vi "test-create-path-trajectory-3-file.vi"() -> ()   [LabVIEW 2019]
uses:
  <vilib>/Rock Robotics/WPI/ThirdParty/MJansen/PathPlanner/TypeDef/PathPlannerTrajectory.ctl
  <vilib>/Rock Robotics/WPI/ThirdParty/MJansen/PathPlanner/TypeDef/PathPlannerTrajectoryState.ctl
  <vilib>/Rock Robotics/WPI/ThirdParty/JAS_Junk/TrajLib/TypeDef/TRANSLATION2D.ctl
  <vilib>/Rock Robotics/WPI/ThirdParty/JAS_Junk/TrajLib/TypeDef/ROTATION2D.ctl
  <vilib>/Rock Robotics/WPI/ThirdParty/MJansen/PathPlanner/TypeDef/PathPlannerPathConstraints.ctl
  <vilib>/Rock Robotics/WPI/ThirdParty/JAS_Junk/TrajLib/TypeDef/TRAJ_STATE.ctl
  <vilib>/Rock Robotics/WPI/ThirdParty/JAS_Junk/TrajLib/TypeDef/POSE2D.ctl
  <vilib>/Rock Robotics/WPI/ThirdParty/JAS_Junk/TrajLib/TypeDef/CHASSIS_SPEEDS.ctl
  <vilib>/Rock Robotics/WPI/ThirdParty/MJansen/PathPlanner/TypeDef/PathPlannerGoalEndState.ctl
  <vilib>/Rock Robotics/WPI/ThirdParty/MJansen/PathPlanner/TypeDef/PathPlannerPath.ctl
  <vilib>/Rock Robotics/WPI/ThirdParty/MJansen/PathPlanner/TypeDef/PathPlannerRotationTarget.ctl
  <vilib>/Rock Robotics/WPI/ThirdParty/MJansen/PathPlanner/TypeDef/PathPlannerConstraintsZone.ctl
  <vilib>/Rock Robotics/WPI/ThirdParty/MJansen/PathPlanner/TypeDef/PathPlannerEventMarker.ctl
  <vilib>/Rock Robotics/WPI/ThirdParty/MJansen/PathPlanner/TypeDef/PathPlannerCommandUtil.ctl
  <vilib>/Rock Robotics/WPI/ThirdParty/MJansen/PathPlanner/ENum/PathPlanner_CommandUtilType_ENUM.ctl
  <vilib>/Rock Robotics/WPI/ThirdParty/MJansen/PathPlanner/TypeDef/PathPlannerPathPoint.ctl
  <vilib>/Rock Robotics/WPI/ThirdParty/MJansen/PathPlanner/TypeDef/PathPlannerWaypoint.ctl
  <vilib>/Rock Robotics/WPI/ThirdParty/MJansen/PathPlanner/TypeDef/PathPlannerPointTowardsZone.ctl
  <vilib>/Rock Robotics/WPI/ThirdParty/MJansen/PathPlanner/TypeDef/PathPlannerIdealStartingState.ctl
  <vilib>/Rock Robotics/WPI/ThirdParty/JAS_Junk/TrajLib/Conv_Deg_Radians.vi
  <vilib>/Rock Robotics/WPI/ThirdParty/JAS_Junk/TrajLib/Rotation2d_CreateAngle.vi
  <vilib>/Rock Robotics/WPI/ThirdParty/MJansen/PathPlanner/VI/PathPlanner_Waypoint_AutoCtrlPoints.vi
  <vilib>/Rock Robotics/WPI/ThirdParty/JAS_Junk/TrajLib/Pose2d_getTranslation.vi
  <vilib>/Rock Robotics/WPI/ThirdParty/JAS_Junk/TrajLib/Pose2d_getRotation.vi
  <vilib>/Rock Robotics/WPI/ThirdParty/JAS_Junk/TrajLib/Translation2d_Minus.vi
  <vilib>/Rock Robotics/WPI/ThirdParty/JAS_Junk/TrajLib/Translation2d_Create_DistAng.vi
  <vilib>/Rock Robotics/WPI/ThirdParty/JAS_Junk/TrajLib/Translation2d_GetDistance.vi
  <vilib>/Rock Robotics/WPI/ThirdParty/MJansen/PathPlanner/VI/PathPlanner_Waypoint_AutoCtrlDistFactor.vi
  <vilib>/Rock Robotics/WPI/ThirdParty/JAS_Junk/TrajLib/Translation2d_Plus.vi
  <vilib>/Rock Robotics/WPI/ThirdParty/JAS_Junk/TrajLib/Translation2d_Create.vi
  <vilib>/Rock Robotics/WPI/ThirdParty/JAS_Junk/TrajLib/Rotation2d_GetAngleCosSin.vi
  <vilib>/Rock Robotics/WPI/ThirdParty/JAS_Junk/TrajLib/Util_CalcDist.vi
  <vilib>/Rock Robotics/WPI/ThirdParty/MJansen/PathPlanner/PathPlanner24.lvlib
  <vilib>/Rock Robotics/WPI/ThirdParty/JAS_Junk/TrajLib/Trajectory_Library.lvlib
  <vilib>/Rock Robotics/WPI/ThirdParty/MJansen/PathPlanner/TypeDef/PathPlannerTrajectoryEvent.ctl
  <vilib>/Rock Robotics/WPI/ThirdParty/MJansen/PathPlanner/TypeDef/PathPlannerTrajectoryEvents.ctl
panel:
  in  "Tab Control":T1(tab)
  in  "Output Trajectory File Name":string="C:\\Shares\\github\\PathPlannerLabVIEW\\PathPlannerSandbox24\\PathPlannerTestPath\\jim1.csv"
  in  "Position 1":T2={"TRANSLATION"={"X"=1.0, "Y"=1.0}, "ROTATION"={"VALUE"=0.0, "COS"=1.0, "SIN"=0.0}} {"ROTATION"."SIN" format="%13.4f"; "ROTATION"."COS" format="%13.4f"; "ROTATION"."VALUE" format="%13.4f"; "TRANSLATION"."Y" format="%14.3f"; "TRANSLATION"."X" format="%14.3f"}
  in  "Position 2":T2={"TRANSLATION"={"X"=1.3, "Y"=1.0}, "ROTATION"={"VALUE"=0.0, "COS"=1.0, "SIN"=0.0}} {"ROTATION"."SIN" format="%13.4f"; "ROTATION"."COS" format="%13.4f"; "ROTATION"."VALUE" format="%13.4f"; "TRANSLATION"."Y" format="%14.3f"; "TRANSLATION"."X" format="%14.3f"}
  in  "Position 3":T2={"TRANSLATION"={"X"=4.0, "Y"=3.7}, "ROTATION"={"VALUE"=1.57, "COS"=0.0, "SIN"=1.0}} {"ROTATION"."SIN" format="%13.4f"; "ROTATION"."COS" format="%13.4f"; "ROTATION"."VALUE" format="%13.4f"; "TRANSLATION"."Y" format="%14.3f"; "TRANSLATION"."X" format="%14.3f"}
  in  "Position 4":T2={"TRANSLATION"={"X"=4.0, "Y"=4.0}, "ROTATION"={"VALUE"=1.57, "COS"=0.0, "SIN"=1.0}} {"ROTATION"."SIN" format="%13.4f"; "ROTATION"."COS" format="%13.4f"; "ROTATION"."VALUE" format="%13.4f"; "TRANSLATION"."Y" format="%14.3f"; "TRANSLATION"."X" format="%14.3f"}
  in  "stop":bool
  in  "StartingSpeeds":T5 {"vOmega" format="%10.3f"; "vY" format="%10.3f"; "vX" format="%10.3f"}
  out "Error":bool
  out "Error 2":bool
  out "PathPlannerConstraints":T6={"MaxVelocityMps;"=0.0, "MaxAccelerationMpsSq;"=0.0, "MaxAngularVelRadPsEc;"=0.0, "MaxAngularAccRadPSecSq"=0.0, "Exists"=FALSE, "Unlimited"=FALSE, "NominalVoltageVolts"=12.0}
  out "GoalEndState":T7={"VelocityMPS"=0.0, "Rotation"={"VALUE"=0.0, "COS"=1.0, "SIN"=0.0}} {"Rotation"."SIN" format="%13.4f"; "Rotation"."COS" format="%13.4f"; "Rotation"."VALUE" format="%13.4f"}
  in  "Angle_Degrees":dbl=90.0
  in  "Velocity":dbl format="%#_13g"
  out "file read\nerror out":errorcluster
  in  "Input Path FileName":string="C:\\Shares\\github\\PathPlannerLabVIEW\\PathPlannerSandbox24\\PathPlannerTestPath\\jim1.path"
  out "write csv file\nerror out":errorcluster
  out "PathPlannerPath":T8={"Reversed"=FALSE, "RotationTargets"=[], "ConstraintZones"=[], "EventMarkers"=[], "GlobalConstraints"={"MaxVelocityMps;"=0.0, "MaxAccelerationMpsSq;"=0.0, "MaxAngularVelRadPsEc;"=0.0, "MaxAngularAccRadPSecSq"=0.0, "Exists"=FALSE, "Unlimited"=FALSE, "NominalVoltageVolts"=1.0}, "GoalEndState"={"VelocityMPS"=0.0, "Rotation"={"VALUE"=0.0, "COS"=1.0, "SIN"=0.0}}, "AllPoints"=[], "Name"="", "Waypoints"=[], "PointTowardsZones"=[], "IdealStartingState"={"VelocityMPS"=0.0, "Rotation"={"VALUE"=0.0, "COS"=1.0, "SIN"=0.0}}, "IsChoreoPath"=FALSE, "PreventFlipping"=FALSE} {"IdealStartingState"."Rotation"."SIN" format="%13.4f"; "IdealStartingState"."Rotation"."COS" format="%13.4f"; "IdealStartingState"."Rotation"."VALUE" format="%13.4f"; "PointTowardsZones"."TargetPosition"."Y" format="%14.3f"; "PointTowardsZones"."TargetPosition"."X" format="%14.3f"; "PointTowardsZones"."RotationOffset"."SIN" format="%13.4f"; "PointTowardsZones"."RotationOffset"."COS" format="%13.4f"; "PointTowardsZones"."RotationOffset"."VALUE" format="%13.4f"; "Waypoints"."nextControl"."Y" format="%14.3f"; "Waypoints"."nextControl"."X" format="%14.3f"; "Waypoints"."anchor"."Y" format="%14.3f"; "Waypoints"."anchor"."X" format="%14.3f"; "Waypoints"."prevControl"."Y" format="%14.3f"; "Waypoints"."prevControl"."X" format="%14.3f"; "AllPoints"."RotationTarget"."rotation"."SIN" format="%13.4f"; "AllPoints"."RotationTarget"."rotation"."COS" format="%13.4f"; "AllPoints"."RotationTarget"."rotation"."VALUE" format="%13.4f"; "AllPoints"."Position"."Y" format="%14.3f"; "AllPoints"."Position"."X" format="%14.3f"; "GoalEndState"."Rotation"."SIN" format="%13.4f"; "GoalEndState"."Rotation"."COS" format="%13.4f"; "GoalEndState"."Rotation"."VALUE" format="%13.4f"; "RotationTargets"."rotation"."SIN" format="%13.4f"; "RotationTargets"."rotation"."COS" format="%13.4f"; "RotationTargets"."rotation"."VALUE" format="%13.4f"}
  out "PathPlannerTrajectory":T18 {"States"."TargetHolonomicRotation"."SIN" format="%13.4f"; "States"."TargetHolonomicRotation"."COS" format="%13.4f"; "States"."TargetHolonomicRotation"."VALUE" format="%13.4f"; "States"."Heading"."SIN" format="%13.4f"; "States"."Heading"."COS" format="%13.4f"; "States"."Heading"."VALUE" format="%13.4f"; "States"."PositionMeters"."Y" format="%14.3f"; "States"."PositionMeters"."X" format="%14.3f"}
  out "outPathPlannerStates":T19[](array[typedef]) {"TargetHolonomicRotation"."SIN" format="%13.4f"; "TargetHolonomicRotation"."COS" format="%13.4f"; "TargetHolonomicRotation"."VALUE" format="%13.4f"; "Heading"."SIN" format="%13.4f"; "Heading"."COS" format="%13.4f"; "Heading"."VALUE" format="%13.4f"; "PositionMeters"."Y" format="%14.3f"; "PositionMeters"."X" format="%14.3f"}
  out "PathPlannerTrajectoryEvents":T20
  in  "Down Button":bool
  in  "Up Button":bool
  in  "index":i32 step=20
  out "LabVIEWStateCount":i32
  out "LabVIEWStates":T22[](array[typedef]) {"POSE"."ROTATION"."SIN" format="%13.4f"; "POSE"."ROTATION"."COS" format="%13.4f"; "POSE"."ROTATION"."VALUE" format="%13.4f"; "POSE"."TRANSLATION"."Y" format="%14.3f"; "POSE"."TRANSLATION"."X" format="%14.3f"}
  out "XY SPLINE":cluster{dbl[], dbl[]}[](graph)
  out "XY Graph":cluster{dbl[], dbl[]}[](graph)
  out "Sample Graph":dbl[][](graph)
  out "LabVIEW Time Plot":cluster{dbl[], dbl[]}[](graph)
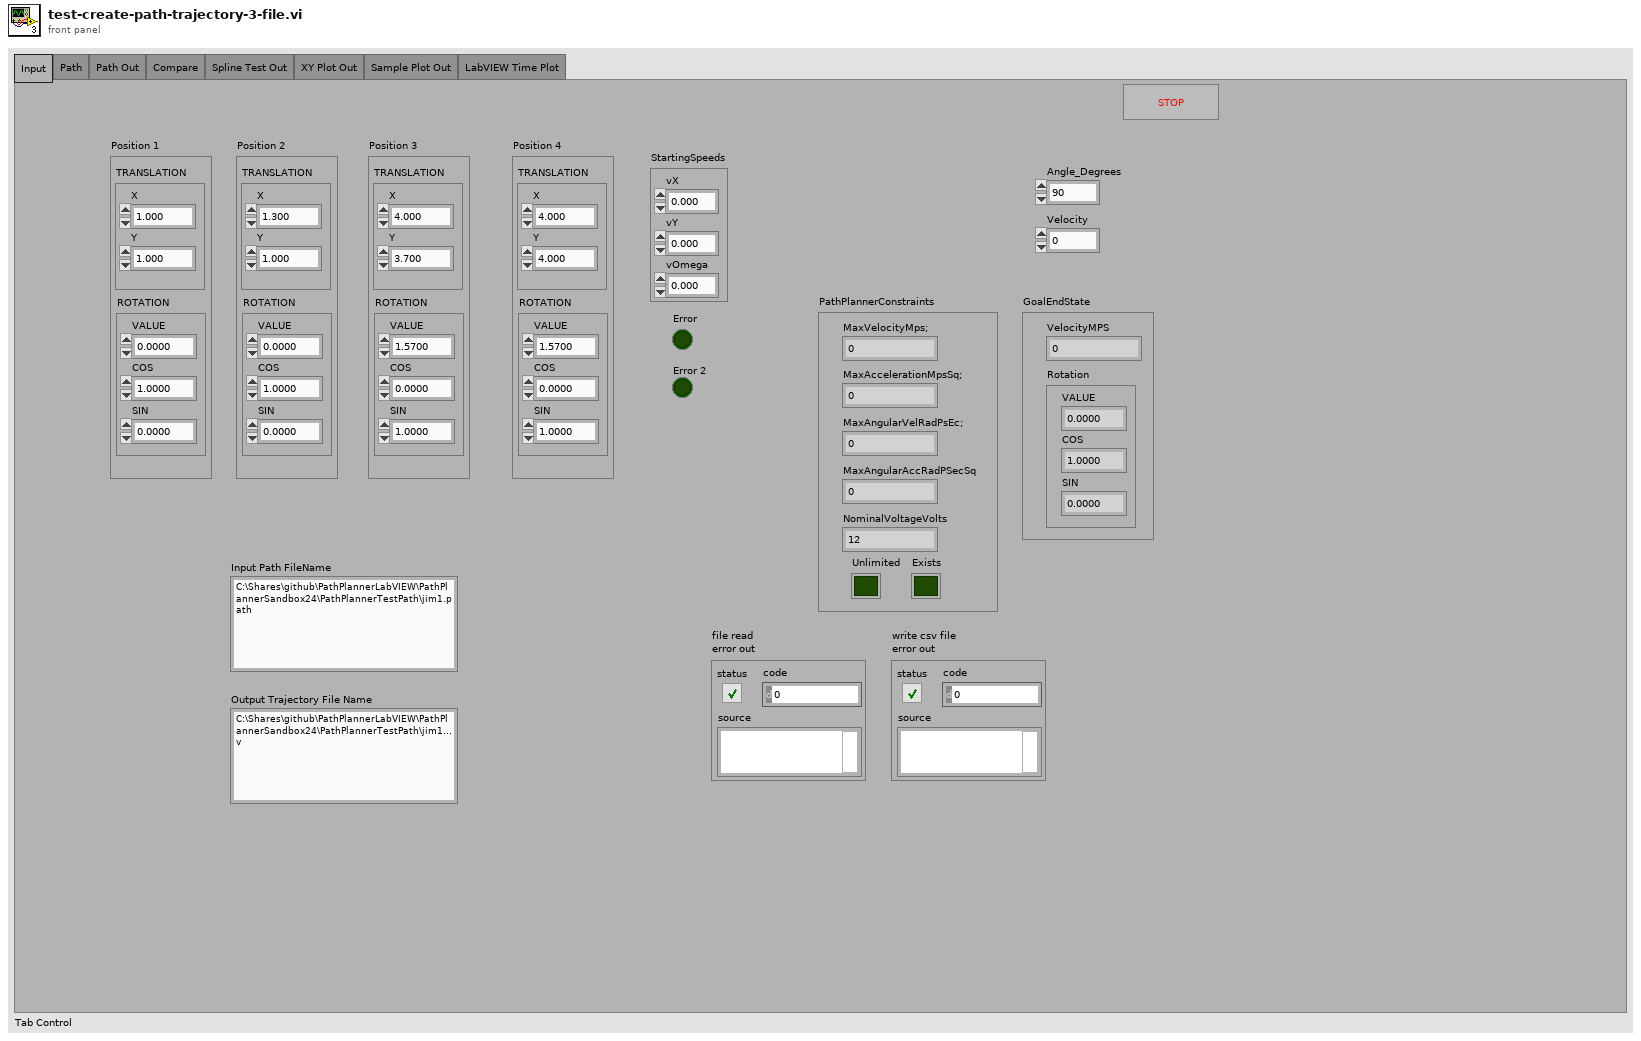
[diagram p1: front panel]
types:
  T1 = enum32{"Input", "Path", "Path Out", "Compare", "Spline Test Out", "XY Plot Out", "Sample Plot Out", "LabVIEW Time Plot"}
  T2 = typedef "Trajectory_Library.lvlib/POSE2D.ctl" = cluster{"TRANSLATION":T3, "ROTATION":T4}
  T3 = typedef "Trajectory_Library.lvlib/TRANSLATION2D.ctl" = cluster{"X":dbl, "Y":dbl}
  T4 = typedef "Trajectory_Library.lvlib/ROTATION2D.ctl" = cluster{"VALUE":dbl, "COS":dbl, "SIN":dbl}
  T5 = typedef "Trajectory_Library.lvlib/CHASSIS_SPEEDS.ctl" = cluster{"vX":dbl, "vY":dbl, "vOmega":dbl}
  T6 = typedef "PathPlanner24.lvlib/PathPlannerPathConstraints.ctl" = cluster{"MaxVelocityMps;":dbl, "MaxAccelerationMpsSq;":dbl, "MaxAngularVelRadPsEc;":dbl, "MaxAngularAccRadPSecSq":dbl, "Exists":bool, "Unlimited":bool, "NominalVoltageVolts":dbl}
  T7 = typedef "PathPlanner24.lvlib/PathPlannerGoalEndState.ctl" = cluster{"VelocityMPS":dbl, "Rotation":T4}
  T8 = typedef "PathPlanner24.lvlib/PathPlannerPath.ctl" = cluster{"Reversed":bool, "RotationTargets":T9[], "ConstraintZones":T10[], "EventMarkers":T11[], "GlobalConstraints":T6, "GoalEndState":T7, "AllPoints":T14[], "Name":string, "Waypoints":T15[], "PointTowardsZones":T16[], "IdealStartingState":T17, "IsChoreoPath":bool, "PreventFlipping":bool}
  T9 = typedef "PathPlanner24.lvlib/PathPlannerRotationTarget.ctl" = cluster{"position":dbl, "rotation":T4, "Exists":bool}
  T10 = typedef "PathPlanner24.lvlib/PathPlannerConstraintsZone.ctl" = cluster{"minPosition":dbl, "maxPosition":dbl, "Constraints":T6, "Present":bool}
  T11 = typedef "PathPlanner24.lvlib/PathPlannerEventMarker.ctl" = cluster{"Position":dbl, "Command":T12, "TriggerName":string, "EndPosition":dbl}
  T12 = typedef "PathPlanner24.lvlib/PathPlannerCommandUtil.ctl" = cluster{"waitTime":dbl, "name":string, "pathName":string, "commands":cluster{"type":T13, "waitTime":dbl, "name":string, "pathName":string}[], "type":T13}
  T13 = typedef "PathPlanner24.lvlib/PathPlanner_CommandUtilType_ENUM.ctl" = enum16{"Unknown", "Wait", "Named", "Path", "Sequential", "Parallel", "Race", "Deadline"}
  T14 = typedef "PathPlanner24.lvlib/PathPlannerPathPoint.ctl" = cluster{"Position":T3, "DistAlongPath":dbl, "MaxV":dbl, "Constraints":T6, "RotationTarget":T9, "WaypointRelativePos":dbl}
  T15 = typedef "PathPlanner24.lvlib/PathPlannerWaypoint.ctl" = cluster{"prevControl":T3, "anchor":T3, "nextControl":T3, "PrevExists":bool, "NextExists":bool}
  T16 = typedef "PathPlanner24.lvlib/PathPlannerPointTowardsZone.ctl" = cluster{"RotationOffset":T4, "Name":string, "TargetPosition":T3, "MinPosition":dbl, "MaxPosition":dbl}
  T17 = typedef "PathPlanner24.lvlib/PathPlannerIdealStartingState.ctl" = cluster{"VelocityMPS":dbl, "Rotation":T4}
  T18 = typedef "PathPlanner24.lvlib/PathPlannerTrajectory.ctl" = cluster{"States":T19[]}
  T19 = typedef "PathPlanner24.lvlib/PathPlannerTrajectoryState.ctl" = cluster{"TimeSeconds":dbl, "VelocityMPS":dbl, "AccerationMpsSq":dbl, "HeadingAngularVelRadPerSec":dbl, "PositionMeters":T3, "Heading":T4, "TargetHolonomicRotation":T4, "CurvatureRadPerMeter":dbl, "PathPlannerConstraints":T6, "DeltaPos":dbl, "WaypointRelPos":dbl}
  T20 = typedef "PathPlanner24.lvlib/PathPlannerTrajectoryEvents.ctl" = cluster{"EventCommands":T21[]}
  T21 = typedef "PathPlanner24.lvlib/PathPlannerTrajectoryEvent.ctl" = cluster{"TimeStampSec":dbl, "CommandUtil":T12}
  T22 = typedef "Trajectory_Library.lvlib/TRAJ_STATE.ctl" = cluster{"TimeSeconds":dbl, "Velocity":dbl, "Acceleration":dbl, "POSE":T2, "Curvature":dbl}
  T23 = typedef "Trajectory_Library.lvlib/TRAJECTORY.ctl" = cluster{"TotalTImeSecs":dbl, "States":T22[]}
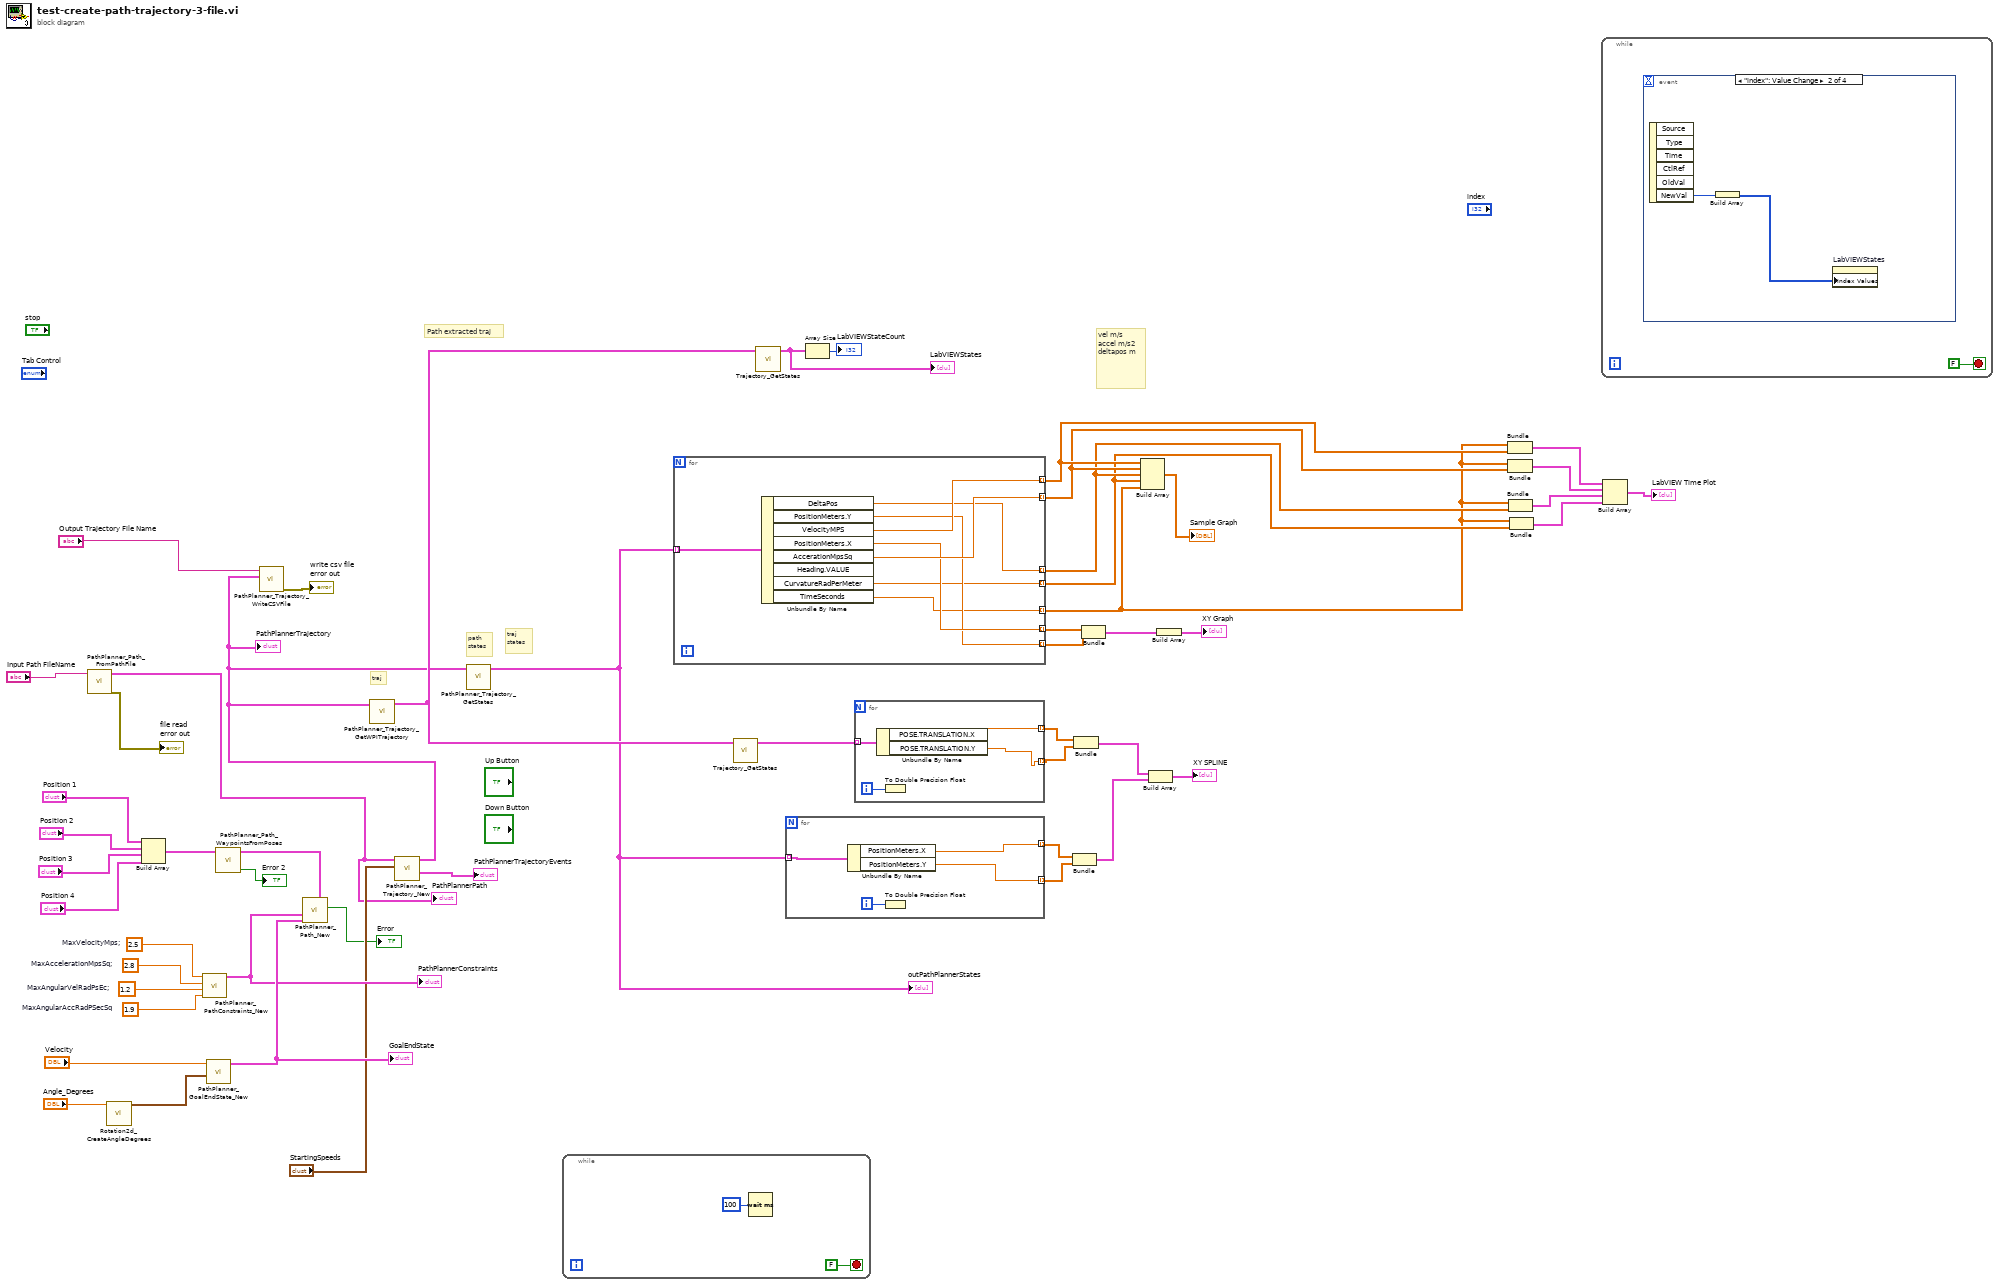
[diagram p0: block diagram]
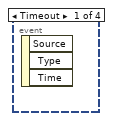
[diagram p2: hidden frame]
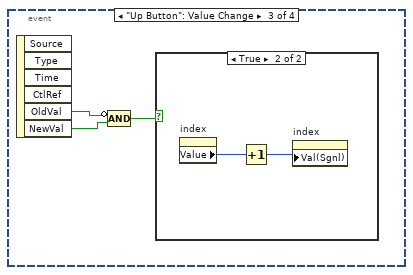
[diagram p3: hidden frame]
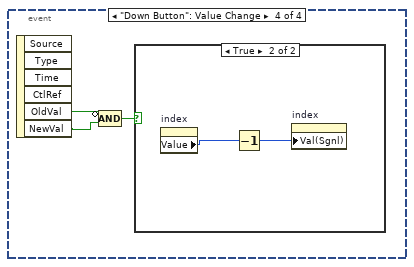
[diagram p5: hidden frame]
diagram:
  w15 = 2.5  # MaxVelocityMps;
  w16 = 2.8  # MaxAccelerationMpsSq;
  w17 = 1.2  # MaxAngularVelRadPsEc;
  w14 = 1.9  # MaxAngularAccRadPSecSq
  # "vel m/s\naccel m/s2\ndeltapos m"
  # "Path extracted traj"
  # "traj"
  # "traj\nstates"
  # "path\nstates"
  n1 = call <vilib>:"PathPlanner_Path_FromPathFile.vi"("FileName"="Input Path FileName") -> ("error out"=→"file read\nerror out":errorcluster, "PathPlannerPath"=w8:T8)  [unwired: 7 in, 2 out]
  "PathPlannerPath" <- w8
  n2 = call <vilib>:"Rotation2d_CreateAngleDegrees.vi"("Angle_Degrees"="Angle_Degrees") -> ("ROTATION"=w9:T4)  [unwired: 10 in]
  n3 = Build Array("Position 1", "Position 2", "Position 3", "Position 4") -> (w21:T2[])
  n4 = call <vilib>:"PathPlanner_PathConstraints_New.vi"("MaxAngularAccRadPSecSq"=w14, "MaxAngularVelRadPsEc;"=w17, "MaxAccelerationMpsSq;"=w16, "MaxVelocityMps;"=w15) -> ("PathPlannerConstraints"=w18:T6)  [unwired: 7 in]
  "PathPlannerConstraints" <- w18
  n5 = call <vilib>:"PathPlanner_GoalEndState_New.vi"("Rotation"=w9, "VelocityMPS"="Velocity") -> ("GoalEndState"=w19:T7)  [unwired: 9 in]
  "GoalEndState" <- w19
  n6 = call <vilib>:"PathPlanner_Path_WaypointsFromPoses.vi"("Poses"=w21) -> ("Error"=→"Error 2":bool, "Waypoints"=w20:T15[])  [unwired: 9 in]
  n7 = call <vilib>:"PathPlanner_Path_New.vi"("Waypoints"=w20, "GoalEndState"=w19, "GlobalConstraints"=w18) -> ("Error"=→"Error":bool)  [unwired: 7 in, 1 out]
  n8 = call <vilib>:"PathPlanner_Trajectory_New.vi"("StartingSpeeds"="StartingSpeeds", "Path"=w8) -> ("PathPlannerTrajectoryEvents"=→"PathPlannerTrajectoryEvents":T20, "PathPlannerTrajectory"=w3:T18)  [unwired: 8 in]
  "PathPlannerTrajectory" <- w3
  n9 = call <vilib>:"PathPlanner_Trajectory_WriteCSVFile.vi"("TRAJECTORY"=w3, "FileName"="Output Trajectory File Name") -> ("error out"=→"write csv file\nerror out":errorcluster)  [unwired: 9 in]
  n10 = call <vilib>:"PathPlanner_Trajectory_GetWPITrajectory.vi"("PathPlannerTrajectory"=w3) -> ("WPI TRAJECTORY"=w39:T23)  [unwired: 9 in, 1 out]
  n11 = call <vilib>:"PathPlanner_Trajectory_GetStates.vi"("PathPlannerTrajectory"=w3) -> ("PathPlannerStates"=w36:T19[])  [unwired: 10 in]
  "outPathPlannerStates" <- w36
  n12 = while {
    stop <- FALSE stop-if-true
    n13 = Wait (ms)(milliseconds to wait=u32 100) -> ()  [unwired: 1 out]
  }
  n14 = for {
    tunnel: [w62] -> w34 mode=indexing
    tunnel: [w61] -> w33 mode=indexing
    tunnel: [w56] -> w32 mode=indexing
    tunnel: [w60] -> w51 mode=indexing
    tunnel: [w59] -> w50 mode=indexing
    tunnel: w36 -> [w58] mode=indexing
    tunnel: [w57] -> w31 mode=indexing
    tunnel: [w55] -> w26 mode=indexing
    n15 = Unbundle By Name(w58) -> ("DeltaPos"=w56:dbl, "PositionMeters.Y"=w59:dbl, "VelocityMPS"=w62:dbl, "PositionMeters.X"=w60:dbl, "AccerationMpsSq"=w61:dbl, "CurvatureRadPerMeter"=w57:dbl, "TimeSeconds"=w55:dbl)  [unwired: 1 out]
  }
  n16 = call <vilib>:"Trajectory_GetStates.vi"("TRAJECTORY"=w39) -> ("States"=w40:T22[])  [unwired: 10 in]
  n17 = call <vilib>:"Trajectory_GetStates.vi"("TRAJECTORY"=w39) -> ("States"=w37:T22[])  [unwired: 10 in]
  "LabVIEWStates" <- w37
  n18 = for {
    tunnel: [w65] -> w45 mode=indexing
    tunnel: w36 -> [w64] mode=indexing
    tunnel: [w63] -> w44 mode=indexing
    i -> [w66]
    n19 = Unbundle By Name(w64) -> ("PositionMeters.X"=w65:dbl, "PositionMeters.Y"=w63:dbl)
    n20 = To Double Precision Float(number=w66) -> ()  [unwired: 1 out]
  }
  n21 = Array Size(array=w37) -> (size(s)=→"LabVIEWStateCount":i32)
  n22 = for {
    tunnel: [w69] -> w47 mode=indexing
    tunnel: [w68] -> w46 mode=indexing
    tunnel: w40 -> [w67] mode=indexing
    i -> [w70]
    n23 = Unbundle By Name(w67) -> ("POSE.TRANSLATION.X"=w69:dbl, "POSE.TRANSLATION.Y"=w68:dbl)
    n24 = To Double Precision Float(number=w70) -> ()  [unwired: 1 out]
  }
  n25 = Bundle(w45, w44) -> (w42:cluster{dbl[], dbl[]})  [unwired: 1 in]
  n26 = Bundle(w47, w46) -> (w43:cluster{dbl[], dbl[]})  [unwired: 1 in]
  n27 = Bundle(w51, w50) -> (w49:cluster{dbl[], dbl[]})  [unwired: 1 in]
  n28 = Build Array(w34, w33, w32, w31, w26) -> (→"Sample Graph":dbl[][])
  n29 = Build Array(w43, w42) -> (→"XY SPLINE":cluster{dbl[], dbl[]}[])
  n30 = Build Array(w49) -> (→"XY Graph":cluster{dbl[], dbl[]}[])
  n31 = Bundle(w26, w34) -> (w30:cluster{dbl[], dbl[]})  [unwired: 1 in]
  n32 = Bundle(w26, w33) -> (w29:cluster{dbl[], dbl[]})  [unwired: 1 in]
  n33 = Bundle(w26, w32) -> (w28:cluster{dbl[], dbl[]})  [unwired: 1 in]
  n34 = Bundle(w26, w31) -> (w27:cluster{dbl[], dbl[]})  [unwired: 1 in]
  n35 = while {
    stop <- FALSE stop-if-true
    n36 = event shown="[1] \"index\": Value Change" {
      selector: _ -> [_ _ _ _]
      dyn-events: _ -> [_ _ _ _]
      timeout: _ -> [_ _ _ _]
      event Timeout {
        n37 = event-data() -> ()  [unwired: 1 in, 3 out]
      }
      event "index": Value Change {
        n38 = event-data() -> ("NewVal"=w73:i32)  [unwired: 1 in, 5 out]
        n39 = Build Array(w73) -> (w72:i32[])
        n40 = property on="LabVIEWStates" class="Arr (strict)"("Index Values"=w72) -> ()  [unwired: 2 in, 2 out]
      }
      event "Up Button": Value Change {
        n41 = event-data() -> ("OldVal"=w76:bool, "NewVal"=w75:bool)  [unwired: 1 in, 4 out]
        n42 = Compound Arithmetic op=AND(invert w76, w75) -> (w74:bool)
        n43 = case shown="True" w74 {
          frame False {
          }
          frame True {
            n44 = property on="index" class="DigNum (strict)"() -> ("Value"=w77:i32)  [unwired: 2 in, 2 out]
            n45 = Increment(x=w77) -> (x+1=w78:i32)
            n46 = property on="index" class="DigNum (strict)"("Val(Sgnl)"=w78) -> ()  [unwired: 2 in, 2 out]
          }
        }
      }
      event "Down Button": Value Change {
        n47 = event-data() -> ("OldVal"=w80:bool, "NewVal"=w79:bool)  [unwired: 1 in, 4 out]
        n48 = Compound Arithmetic op=AND(invert w80, w79) -> (w81:bool)
        n49 = case shown="True" w81 {
          frame False {
          }
          frame True {
            n50 = property on="index" class="DigNum (strict)"() -> ("Value"=w82:i32)  [unwired: 2 in, 2 out]
            n51 = Decrement(x=w82) -> (x-1=w83:i32)
            n52 = property on="index" class="DigNum (strict)"("Val(Sgnl)"=w83) -> ()  [unwired: 2 in, 2 out]
          }
        }
      }
    }
  }
  n53 = Build Array(w30, w29, w28, w27) -> (→"LabVIEW Time Plot":cluster{dbl[], dbl[]}[])
